vi "finishUp.vi"(8 "error in (no error)":errorcluster, 11 "BECHWCBasic in":refnum<class "BECHWCBasic.lvclass">) -> (0 "error out":errorcluster, 3 "BECHWCBasic out":refnum<class "BECHWCBasic.lvclass">)   [LabVIEW 2009, in "Hardware.lvlib" / "HWControllers.lvlib" / "BECHWCBasic.lvclass"]
uses:
  BECHWCBasic.lvclass
  HWController.lvclass
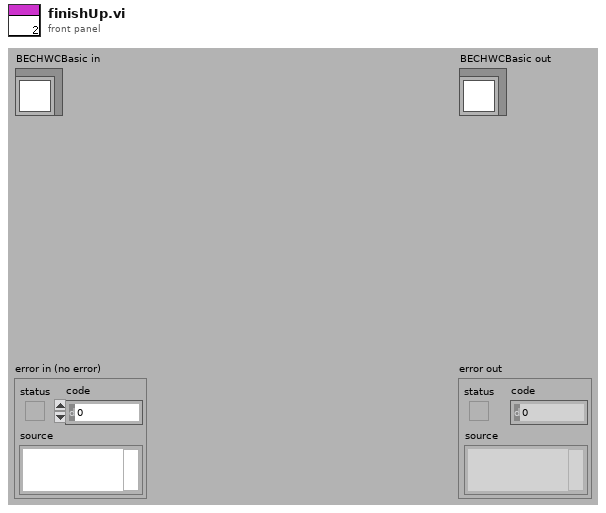
[diagram p1: front panel]
types:
  T1 = enum16{"Ready", "Compiling", "Configured", "Running", "Stopping", "Unresolved Error"}
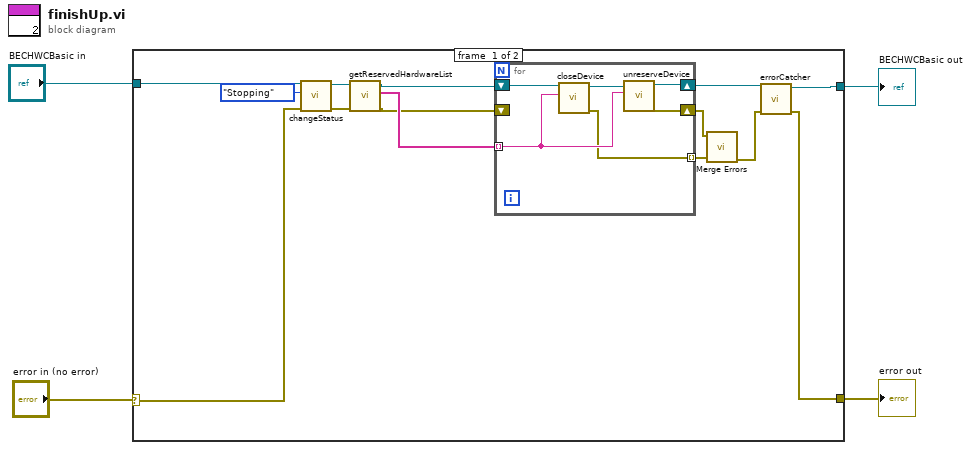
[diagram p0: block diagram]
diagram:
  n1 = case shown="No Error" "error in (no error)" {
    selector: "error in (no error)" -> [w14 w25]
    tunnel: "BECHWCBasic in" -> [w17 w26]
    tunnel: [w6 w26] -> w2
    tunnel: [w5 w25] -> w1
    frame #0 {
      n2 = call "changeStatus.vi"("error in (no error)"=w14, "status"=T1."Stopping", "HWController in"=w17) -> ("error out"=w15:errorcluster, "HWController out"=w16:refnum<class "BECHWCBasic.lvclass">)  [unwired: 7 in]
      n3 = call "getReservedHardwareList.vi"("error in (no error)"=w15, "HWController.lvclass in"=w16) -> ("error out"=w12:errorcluster, "reservedHardwareList"=w18:string[], "HWController.lvclass out"=w13:refnum<class "BECHWCBasic.lvclass">)  [unwired: 7 in]
      n4 = for {
        shift-right: [w22] -> w8
        shift-left: w13 -> [w24]
        shift-right: [w21] -> w10
        shift-left: w12 -> [_]
        tunnel: w18 -> [w20] mode=indexing
        tunnel: [w19] -> w11 mode=indexing
        n5 = call "closeDevice.vi"("deviceName"=w20, "BECHWCBasic in"=w24) -> ("error out"=w19:errorcluster, "BECHWCBasic out"=w23:refnum<class "BECHWCBasic.lvclass">)  [unwired: 8 in]
        n6 = call "unreserveDevice.vi"("deviceName"=w20, "HWController.lvclass in"=w23) -> ("error out"=w21:errorcluster, "HWController.lvclass out"=w22:refnum<class "BECHWCBasic.lvclass">)  [unwired: 8 in]
      }
      n7 = call <vilib>:"Merge Errors.vi"("error array in"=w11, "error in 1 (no error)"=w10) -> ("error out"=w7:errorcluster)  [unwired: 5 in]
      n8 = call-dynamic "errorCatcher.vi"("error in (no error)"=w7, "HWController in"=w8) -> ("error out"=w5:errorcluster, "HWController out"=w6:refnum<class "BECHWCBasic.lvclass">)  [unwired: 8 in]
    }
    frame #1 {
    }
  }
  "error out" <- w1
  "BECHWCBasic out" <- w2
